vi "Draw End Program Status.vi"(10 "Data Type":T1, 11 "Program Status String":string) -> (1 "Purging_Match":i16, 2 "Power_Match":i16, 3 "Draw_Match":i16, 4 "StartingDrawafterCutout_Match":i16)   [LabVIEW 2023]
uses:
  Type Definitions/HEWH Meter Type.ctl
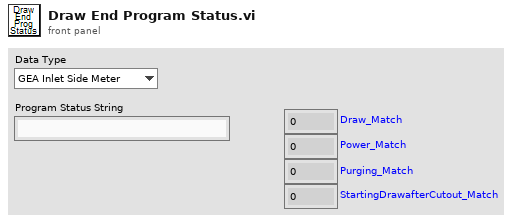
[diagram p1: front panel]
types:
  T1 = typedef "HEWH Meter Type.ctl" = enum16{"GEA Inlet Side Meter", "GEA Outlet Side Meter", "CSA Inlet Side Meter"}
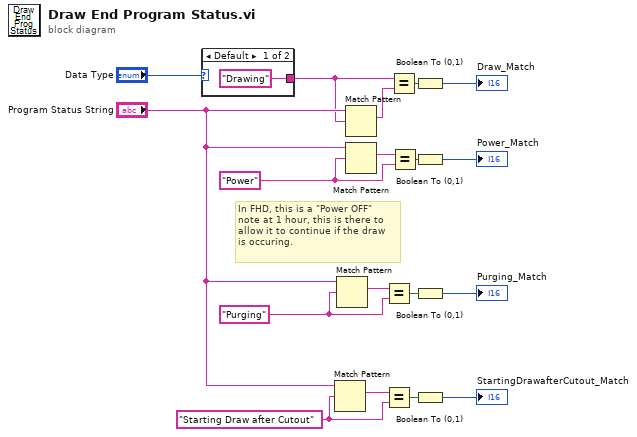
[diagram p0: block diagram]
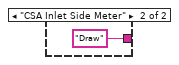
[diagram p2: hidden frame]
diagram:
  w8 = "Starting Draw after Cutout"
  w7 = "Purging"
  w2 = "Power"
  # "In FHD, this is a \"Power OFF\"\nnote at 1 hour, this is there to\nallow it to continue if the draw\nis occuring."
  n1 = case shown="Default" "Data Type" {
    tunnel: ["Drawing" "Draw"] -> w5
    frame Default {
    }
    frame "CSA Inlet Side Meter" {
    }
  }
  n2 = Match Pattern(string="Program Status String", regular expression=w8) -> (match substring=w9:string)  [unwired: 1 in, 3 out]
  n3 = Match Pattern(string="Program Status String", regular expression=w7) -> (match substring=w6:string)  [unwired: 1 in, 3 out]
  n4 = Match Pattern(string="Program Status String", regular expression=w5) -> (match substring=w1:string)  [unwired: 1 in, 3 out]
  n5 = Match Pattern(string="Program Status String", regular expression=w2) -> (match substring=w3:string)  [unwired: 1 in, 3 out]
  n6 = Equal?(x=w6, y=w7) -> (x = y?=w17:bool)
  n7 = Equal?(x=w9, y=w8) -> (x = y?=w18:bool)
  n8 = Equal?(x=w5, y=w1) -> (x = y?=w12:bool)
  n9 = Equal?(x=w3, y=w2) -> (x = y?=w16:bool)
  n10 = Boolean To (0,1)(Boolean=w12) -> (0, 1=→"Draw_Match":i16)
  n11 = Boolean To (0,1)(Boolean=w16) -> (0, 1=→"Power_Match":i16)
  n12 = Boolean To (0,1)(Boolean=w17) -> (0, 1=→"Purging_Match":i16)
  n13 = Boolean To (0,1)(Boolean=w18) -> (0, 1=→"StartingDrawafterCutout_Match":i16)
